vi "RichToFlatni_xnet_can_bm_api_SetStreamingFilterRequest.vi"(5 "OutputClusterType":T1, 11 "InputCluster":T6) -> (3 "OutputCluster":T1)   [LabVIEW 2025, in "xnet_can_bus_monitor_api_client.lvlib"]
uses:
  xnet_can_bus_monitor_api_client.lvlib
  ni_xnet_can_bm_api_SetStreamingFilterRequest.ctl
  ni_xnet_can_bm_api_Session.ctl
  ni_xnet_can_bm_api_FilterInfo.ctl
  ni_xnet_can_bm_api_DirectionFilter.ctl
  ni_xnet_can_bm_api_FrameFilter.ctl
  ni_xnet_can_bm_api_SetStreamingFilterRequest_Flat.ctl
  ni_xnet_can_bm_api_Session_Flat.ctl
  ni_xnet_can_bm_api_FilterInfo_Flat.ctl
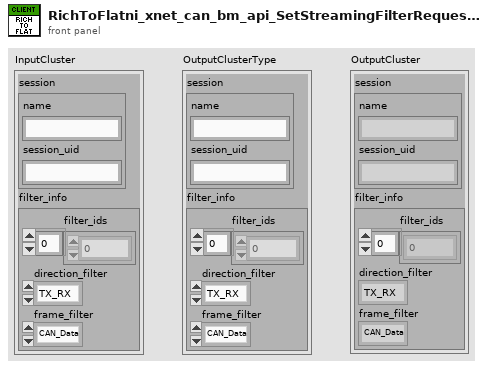
[diagram p1: front panel]
types:
  T1 = typedef "xnet_can_bus_monitor_api_client.lvlib/ni_xnet_can_bm_api_SetStreamingFilterRequest_Flat.ctl" = cluster{"session":T2, "filter_info":T3}
  T2 = typedef "xnet_can_bus_monitor_api_client.lvlib/ni_xnet_can_bm_api_Session_Flat.ctl" = cluster{"name":string, "session_uid":string}
  T3 = typedef "xnet_can_bus_monitor_api_client.lvlib/ni_xnet_can_bm_api_FilterInfo_Flat.ctl" = cluster{"filter_ids":u32[], "direction_filter":T4, "frame_filter":T5}
  T4 = typedef "xnet_can_bus_monitor_api_client.lvlib/ni_xnet_can_bm_api_DirectionFilter.ctl" = enum32{"TX_RX", "RX", "TX"}
  T5 = typedef "xnet_can_bus_monitor_api_client.lvlib/ni_xnet_can_bm_api_FrameFilter.ctl" = enum32{"CAN_Data", "CAN_Remote", "CAN_Bus_Error", "CAN_2_Data", "CAN_FD_Data", "CAN_FD_BRS_Data", "J1939_Data", "Delay", "Log_Trigger", "Start_Trigger", "All"}
  T6 = typedef "xnet_can_bus_monitor_api_client.lvlib/ni_xnet_can_bm_api_SetStreamingFilterRequest.ctl" = cluster{"session":T7, "filter_info":T8}
  T7 = typedef "xnet_can_bus_monitor_api_client.lvlib/ni_xnet_can_bm_api_Session.ctl" = cluster{"name":string, "session_uid":string}
  T8 = typedef "xnet_can_bus_monitor_api_client.lvlib/ni_xnet_can_bm_api_FilterInfo.ctl" = cluster{"filter_ids":u32[], "direction_filter":T4, "frame_filter":T5}
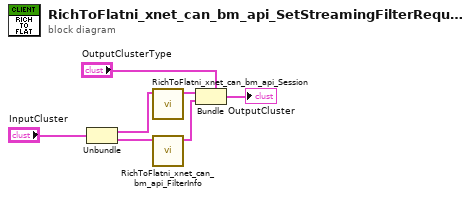
[diagram p0: block diagram]
diagram:
  n1 = Unbundle "Unbundle"("InputCluster") -> ("session"=w4:T7, "filter_info"=w2:T8)
  n2 = call "RichToFlatni_xnet_can_bm_api_Session.vi"("InputCluster"=w4) -> ("OutputCluster"=w3:T2)  [unwired: 10 in]
  n3 = call "RichToFlatni_xnet_can_bm_api_FilterInfo.vi"("InputCluster"=w2) -> ("OutputCluster"=w1:T3)  [unwired: 10 in]
  n4 = Bundle "Bundle"(cluster="OutputClusterType", "session"=w3, "filter_info"=w1) -> (→"OutputCluster":T1)
